vi "Keyence.TuningSequence.vi"(6 "Timeout [ms] (1000)":i32=1000, 7 "Bank":i32, 8 "error in":errorcluster) -> (0 "error out":errorcluster, 2 "Tuned?":bool)   [LabVIEW 2015]
uses:
  Keyence.Cmd.ParametersBank.ctl
  Keyence.Cmd.OperationCommands.ctl
panel:
  # "b1 - 0560010006000450\nb2 - 0480010005800450\nb3 - 0400010005000450\nb4 - 0320010004200450\nb5 - 0235060003350800\nb6 - 0150060002500800"
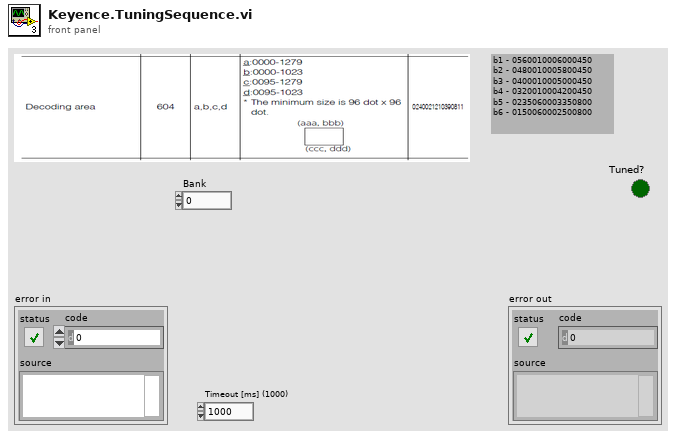
[diagram p1: front panel]
types:
  T1 = typedef "Keyence.Cmd.ParametersBank.ctl" = enum16{"Decoding Area", "Scan.DynamicRange"}
  T2 = typedef "Keyence.Cmd.OperationCommands.ctl" = enum16{"Area limit"}
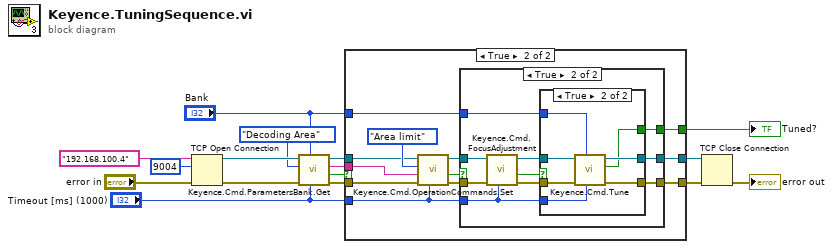
[diagram p0: block diagram]
diagram:
  n1 = TCP Open Connection(address="192.168.100.4", remote port or service name=u16 9004, error in (no error)="error in") -> (connection ID=w13:refnum<k5>, error out=w12:errorcluster)  [unwired: 2 in]
  n2 = call "Keyence.Cmd.ParametersBank.Get.vi"("Timeout [ms] (1000)"="Timeout [ms] (1000)", "Bank"="Bank", "error in"=w12, "Cmd"=Keyence.Cmd.ParametersBank."Decoding Area", "cID in"=w13) -> ("error out"=w9:errorcluster, "OK?"=w7:bool, "Response"=w8:string, "cID out"=w10:refnum<k5>)  [unwired: 3 in]
  n3 = case shown="True" w7 {
    tunnel: [w17 w30] -> w5
    tunnel: [w18 w29] -> w4
    tunnel: "Timeout [ms] (1000)" -> [_ w25]
    tunnel: w10 -> [w18 w24]
    tunnel: w9 -> [w17 w23]
    tunnel: w8 -> [_ w22]
    tunnel: "Bank" -> [_ w20]
    tunnel: [_ w19] -> w3
    frame False {
    }
    frame True {
      n4 = call "Keyence.Cmd.OperationCommands.Set.vi"("Timeout [ms] (1000)"=w25, "error in"=w23, "Parameters"=w22, "Cmd"=Keyence.Cmd.OperationCommands."Area limit", "cID in"=w24) -> ("error out"=w27:errorcluster, "OK?"=w21:bool, "cID out"=w26:refnum<k5>)  [unwired: 3 in, 1 out]
      n5 = case shown="True" w21 {
        tunnel: [w31 w34] -> w30
        tunnel: [w32 w35] -> w29
        tunnel: w27 -> [w31 w42]
        tunnel: w26 -> [w32 w41]
        tunnel: w25 -> [_ w36]
        tunnel: w20 -> [_ w37]
        tunnel: [_ w33] -> w19
        frame False {
        }
        frame True {
          n6 = call "Keyence.Cmd.FocusAdjustment.vi"("Timeout [ms] (1000)"=w36, "error in"=w42, "cID in"=w41) -> ("error out"=w38:errorcluster, "OK?"=w39:bool, "cID out"=w40:refnum<k5>)  [unwired: 5 in, 1 out]
          n7 = case shown="True" w39 {
            tunnel: w40 -> [w44 w51]
            tunnel: w38 -> [w43 w50]
            tunnel: w37 -> [_ w49]
            tunnel: w36 -> [_ w48]
            tunnel: [w44 w47] -> w35
            tunnel: [w43 w46] -> w34
            tunnel: [_ w45] -> w33
            frame False {
            }
            frame True {
              n8 = call "Keyence.Cmd.Tune.vi"("Timeout [ms] (1000)"=w48, "Bank"=w49, "error in (no error)"=w50, "cID in"=w51) -> ("error out"=w46:errorcluster, "Tune succeded"=w45:bool, "cID out"=w47:refnum<k5>)  [unwired: 4 in, 1 out]
            }
          }
        }
      }
    }
  }
  "Tuned?" <- w3
  n9 = TCP Close Connection(connection ID=w4, error in (no error)=w5) -> (error out=→"error out":errorcluster)  [unwired: 1 in, 1 out]
